vi "Generate Report.vi"(8 "error in (no error)":errorcluster, 11 "Slideshow Report in":refnum<class "Slideshow Report.lvclass">) -> (0 "error out":errorcluster, 3 "Slideshow Report out":refnum<class "Slideshow Report.lvclass">)   [LabVIEW 2020, in "Slideshow Report.lvclass"]
uses:
  Slideshow Report.lvclass
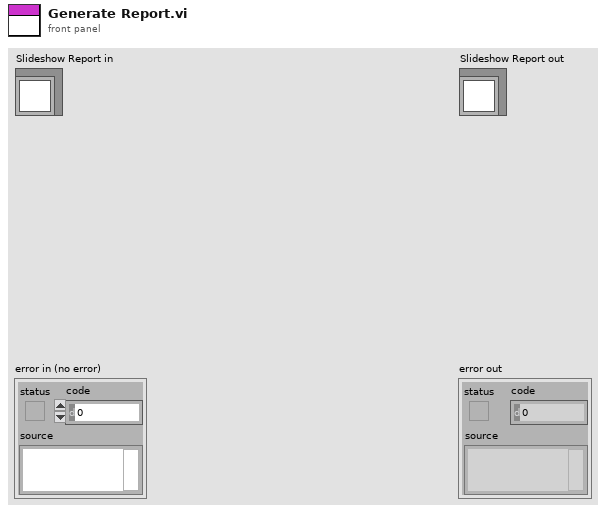
[diagram p1: front panel]
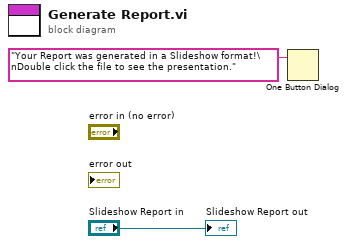
[diagram p0: block diagram]
diagram:
  n1 = One Button Dialog(message="Your Report was generated in a Slideshow format!\nDouble click the file to see the presentation.") -> ()  [unwired: 1 in, 1 out]
  "Slideshow Report out" <- "Slideshow Report in"
